vi "Semaphore Create Object.vi"(8 "error in (no error)":errorcluster, 11 "semaphore pointer":u64) -> (0 "error out":errorcluster, 3 "Semaphore out":T1)   [LabVIEW 2016, in "Linux RT IPC.POSIX Threads.lvlib" / "Semaphore.lvclass"]
doc: "Creates a LabVIEW object used to encapsulate a semaphore object referenced by semaphore pointer."
uses:
  Semaphore.lvclass
  Controls/reference.ctl
  C:/Git/SourceTree/LinuxRT-IPC/Source/POSIX Threads/Classes/POSIX Thread Object/POSIX Thread Object.lvclass
  POSIX Thread Object/POSIX Thread Object.lvclass/POSIX Thread Object.ctl
  POSIX Thread Object/POSIX Thread Object.lvclass
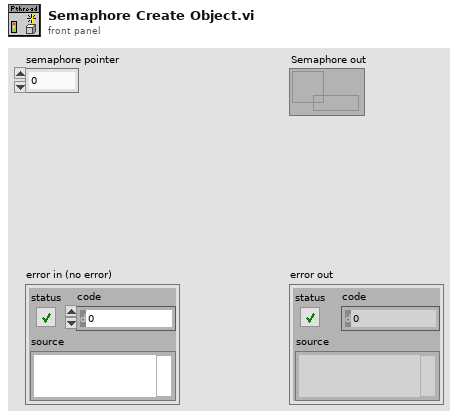
[diagram p1: front panel]
types:
  T1 = typedef "Linux RT IPC.POSIX Threads.lvlib/Semaphore.lvclass/reference.ctl" = refnum<data-value>
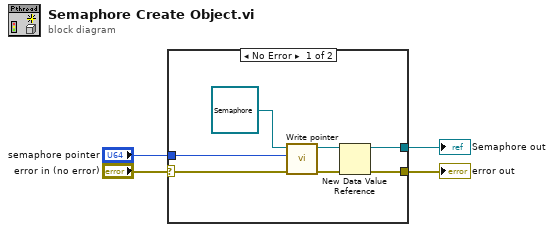
[diagram p0: block diagram]
diagram:
  n1 = case shown="No Error" "error in (no error)" {
    selector: "error in (no error)" -> [w11 w12]
    tunnel: [w6 w12] -> w3
    tunnel: "semaphore pointer" -> [w10 _]
    tunnel: [w5 _] -> w1
    frame No Error {
      n2 = call "Write pointer.vi"("error in (no error)"=w11, "pointer"=w10, "POSIX Thread Object in"=refnum<class "Semaphore.lvclass"> refnum ("POSIX Threads.lvlib:Semaphore")) -> ("error out"=w8:errorcluster, "POSIX Thread Object out"=w7:refnum<class "Semaphore.lvclass">)  [unwired: 7 in]
      n3 = New Data Value Reference(data value=w7, error in=w8) -> (data value reference=w5:refnum<data-value>, error out=w6:errorcluster)
    }
    frame Error {
    }
  }
  "error out" <- w3
  "Semaphore out" <- w1
